vi "RoomAlert.vi"() -> ()   [LabVIEW 2018, in "Visualization.lvlib" / "VisualizeSensor.lvclass"]
doc: "This VI listens for any measurement data associated with the provided PluginName and displays it to the user for analysis. The display is only suitable for data coming from the RoomAlert Plugin."
uses:
  VisualizeSensor.lvclass
  Sensor/SensorShared/clSensorData.ctl
  <vilib>/event_ctls.llb/usereventprio.ctl
  VisualizeBase/VisualizeBase_class/Requests/VisUserEventType.ctl
  <extravilib>/ChannelInstances/Tag-bool/Write With Abort.vi
  <extravilib>/ChannelInstances/Tag-bool/Read With Abort.vi
  <extravilib>/ChannelInstances/Tag-bool/Instantiate.vi
  <extravilib>/ChannelInstances/Tag-bool/EndpointRead.vi
  <vilib>/Utility/error.llb/Error Cluster From Error Code.vi
  <extravilib>/ChannelInstances/Tag-bool/Endpoint.vi
  <vilib>/ErrorRing/Error Ring.xnode
  <userlib>/NIST/NISTErrorLib/NISTErrorLib.lvlib
  VisualizeBase/VisualizeBase_class/VisualizeBase.lvclass
  Sensor/SensorShared/SensorShared.lvlib
  Sensor/SensorModule/SensorModule.lvlib
  <extravilib>/ChannelInstances/Tag-bool.lvlib
  TestClass/Test.lvclass
panel:
  in  "ModuleID":i32
  in  "Log Data":bool=TRUE
  in  "btnStop":bool
  in  "btnReset":bool
  in  "btnClearTest":bool
  out "RoomAlert":waveform(dbl)[](graph)=[{"t0"=timestamp(3657200531.6397257 s since 1904-01-01), "dt"=1.0, "Y"=[46.19]}, {"t0"=timestamp(3657200531.6397257 s since 1904-01-01), "dt"=1.0, "Y"=[2.0]}, {"t0"=timestamp(3657200531.6397257 s since 1904-01-01), "dt"=1.0, "Y"=[60.0]}]
  out "LightTower":T1
  out "ErrorArray":errorcluster[](array[cluster])
  out "Incorrect DataType?":bool
  out "String Results":string="Sensor.RoomAlert1"
  in  "PluginName":string="Sensor.RoomAlert1"
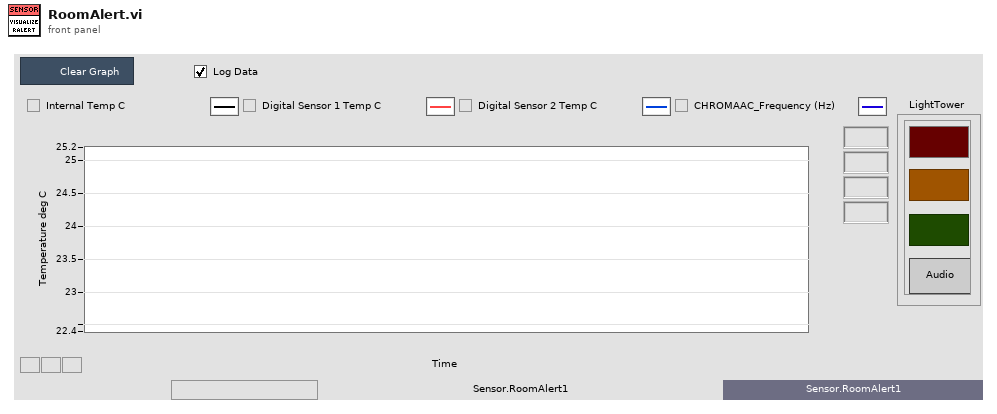
[diagram p1: front panel]
types:
  T1 = cluster{"Red":bool, "Amber":bool, "Green":bool, "Audio":bool}
  T2 = enum16{"open", "open or create", "create or replace", "create", "open (read-only)"}
  T3 = typedef "Visualization.lvlib/VisualizeBase.lvclass/VisRequestEvents.ctl" = cluster{"StopRequest":refnum<user-event>, "ResetRequest":refnum<user-event>, "FP Pop In or Out":refnum<user-event>}
  T4 = typedef "SensorShared.lvlib/clBroadcastEvents.ctl" = cluster{"DidInit":refnum<user-event>, "StatusUpdate":refnum<user-event>, "ErrorReport":refnum<user-event>, "DidStop":refnum<user-event>, "PathToINI":refnum<user-event>, "SensorReport":refnum<user-event>, "SensorConfig":refnum<user-event>}
  T5 = typedef "SensorShared.lvlib/clSensorData.ctl" = cluster{"SensorType":string, "SensorData":variant}
  T6 = typedef "Visualization.lvlib/VisualizeBase.lvclass/VisUserEventType.ctl" = cluster{"BusIndex":i8, "Data":variant}
  T7 = typedef "usereventprio.ctl" = enum32{"high priority", "normal priority"}
  T8 = cluster{"Red":bool, "Amber":bool, "Green":bool, "Audio":bool}[]
  T9 = typedef "Tag-bool.lvlib/))Channel.ctl" = refnum<queue>
  T10 = typedef "sizeaction.ctl" = enum32{"Minimized", "Maximized", "Resized"}
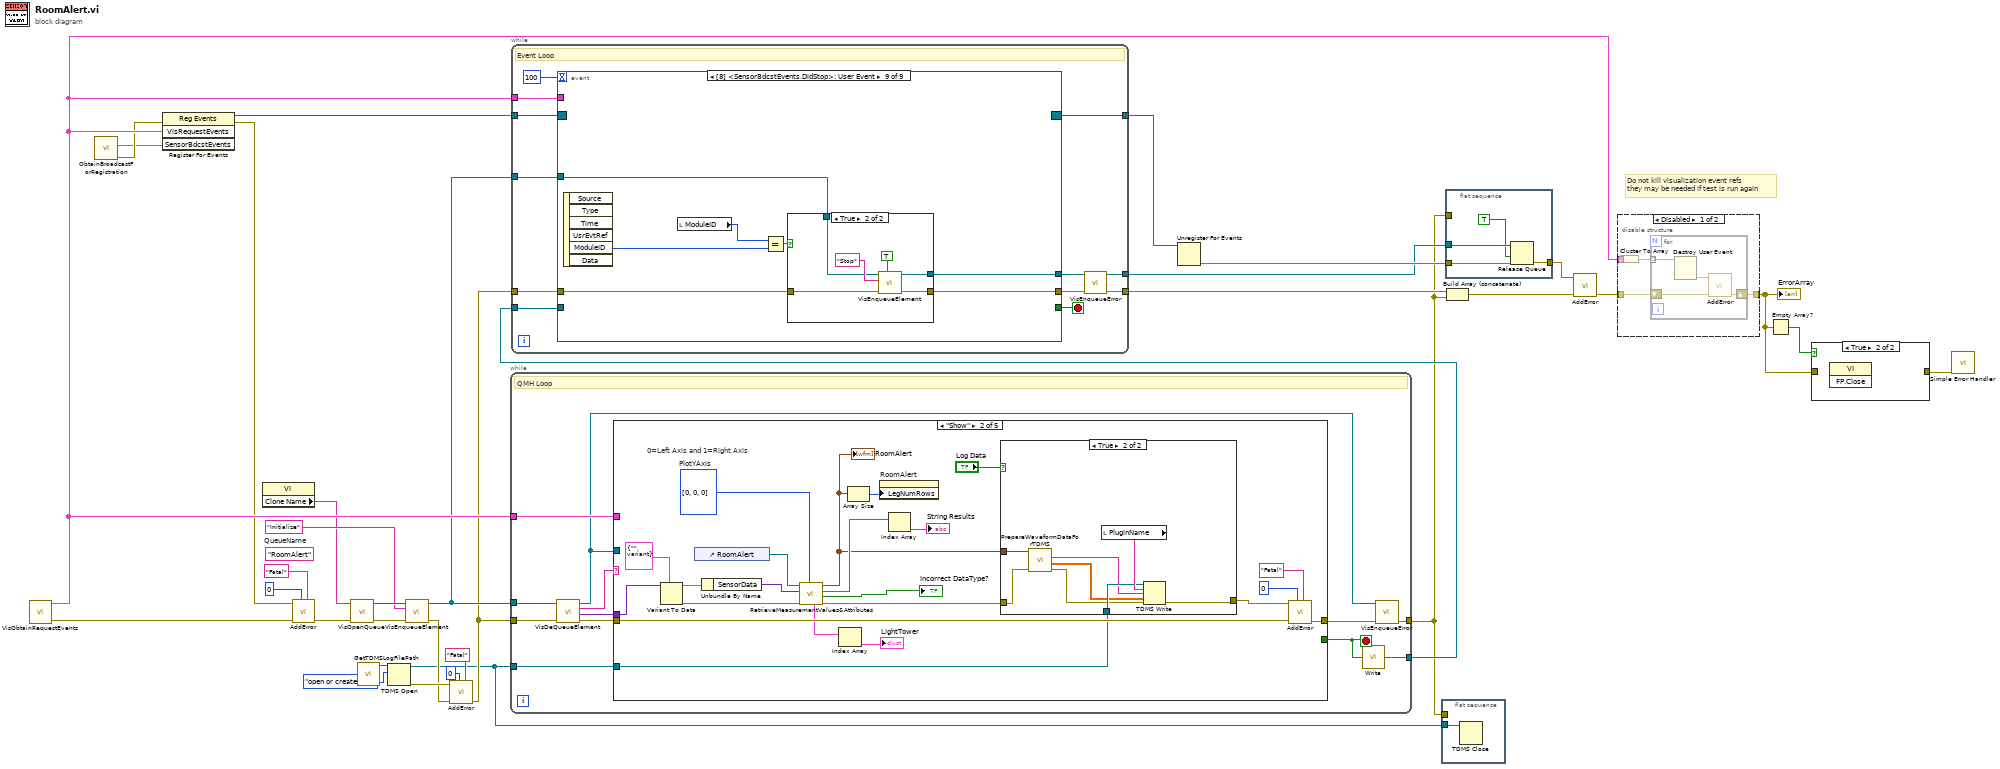
[diagram p0: block diagram]
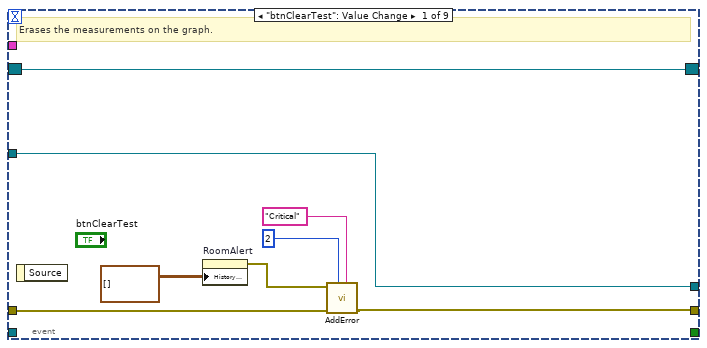
[diagram p3: hidden frame]
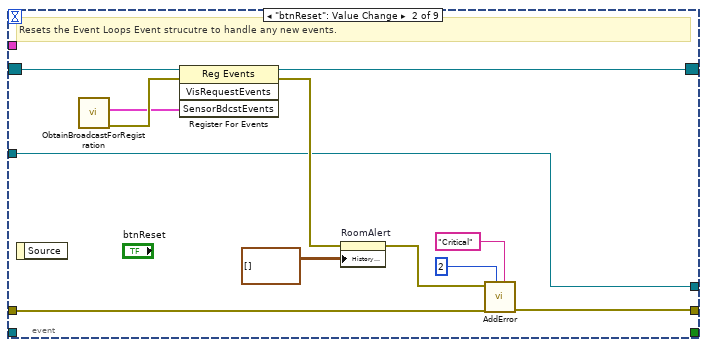
[diagram p4: hidden frame]
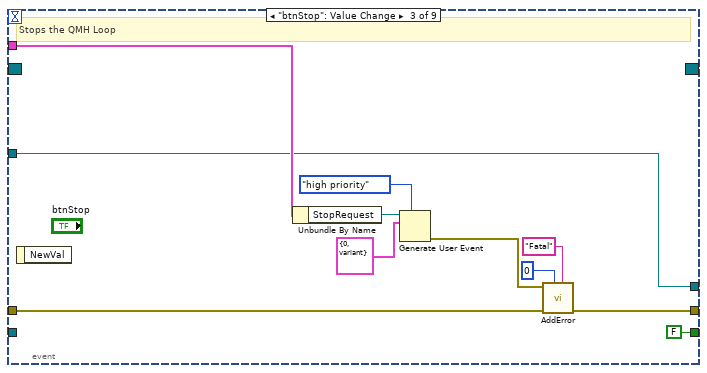
[diagram p5: hidden frame]
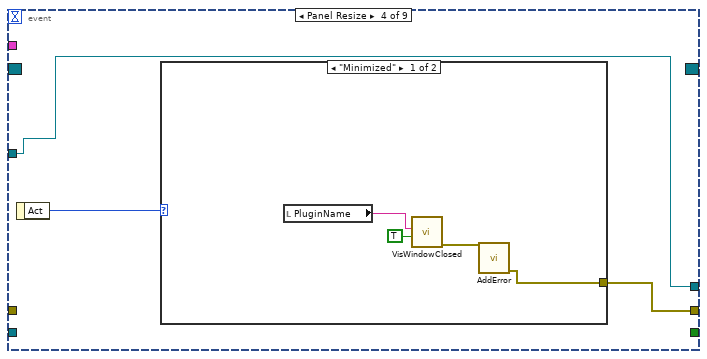
[diagram p6: hidden frame]
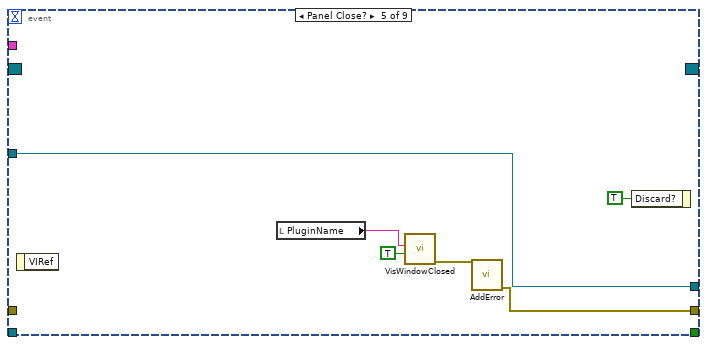
[diagram p8: hidden frame]
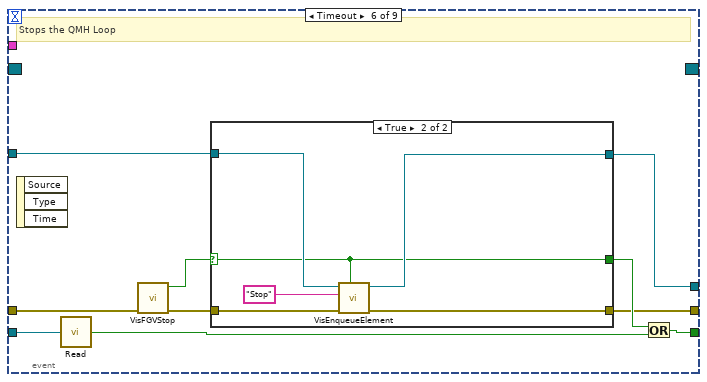
[diagram p9: hidden frame]
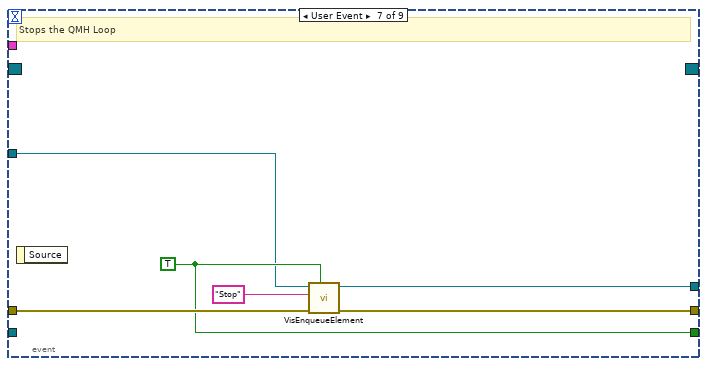
[diagram p11: hidden frame]
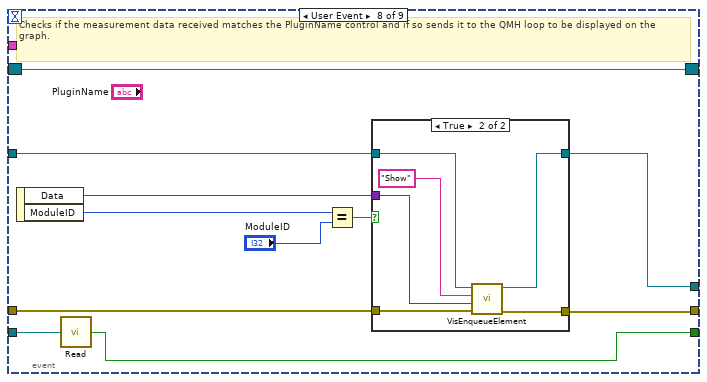
[diagram p12: hidden frame]
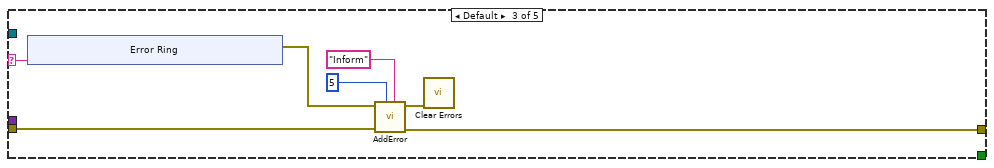
[diagram p17: hidden frame]
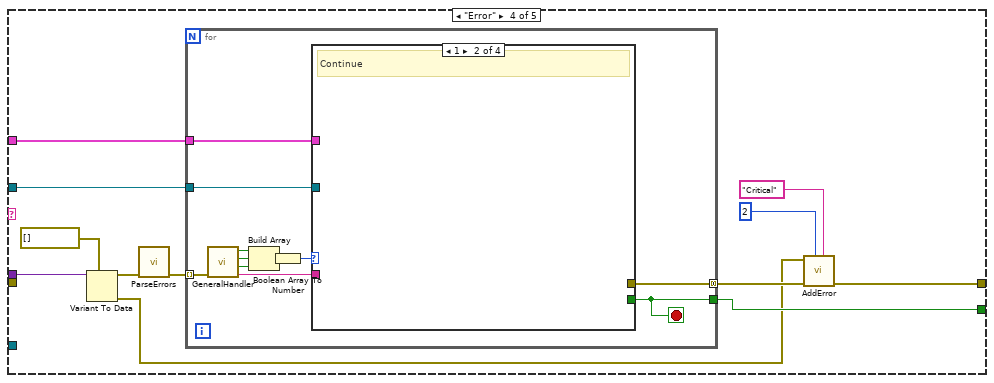
[diagram p18: hidden frame]
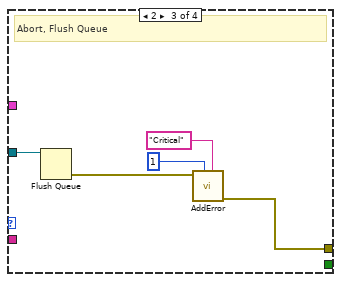
[diagram p20: hidden frame]
diagram:
  (unwired) "RoomAlert"  # QueueName
  # "Do not kill visualization event refs\nthey may be needed if test is run again"
  n1 = call "VisObtainRequestEvents.vi"() -> ("Error"=w25:errorcluster[], "VisRequestEvents"=w27:T3)  [unwired: 10 in]
  n2 = call "ObtainBroadcastForRegistration.vi"() -> ("error out"=w21:errorcluster, "SensorBdcstEvents"=w12:T4)  [unwired: 10 in]
  n3 = register-events(error in=w21, w27, w12) -> (reference out=w34:refnum<event-registration>, error out=w24:errorcluster)  [unwired: 1 in]
  n4 = property class="VI"() -> ("Clone Name"=w10:string)  [unwired: 2 in, 2 out]
  n5 = call <userlib>:"AddError.vi"("Severity"="Fatal", "Priority"=u8 0, "ErrorArray In"=w25, "error in (no error)"=w24) -> ("ErrorArray Out"=w20:errorcluster[])  [unwired: 6 in, 1 out]
  n6 = call "VisOpenQueue.vi"("Error Array In"=w20, "QueueName"=w10) -> ("Error Array Out"=w18:errorcluster[], "queue out"=w19:refnum<queue>)  [unwired: 8 in]
  n7 = call "GetTDMSLogFilePath.vi"() -> ("TDMS Log File Path"=w9:path)  [unwired: 11 in]
  n8 = TDMS Open(10:T2."open or create" ("operation (0:open)"), 11:w9) -> (0:w6:errorcluster, 3:w2:refnum<k34>)  [unwired: 5 in]
  n9 = call "VisEnqueueElement.vi"("Error Array In"=w18, "Message"="Initialize", "queue in"=w19) -> ("Error Array Out"=w5:errorcluster[], "queue out"=w16:refnum<queue>)  [unwired: 7 in]
  n10 = call <userlib>:"AddError.vi"("Severity"="Fatal", "Priority"=u8 0, "ErrorArray In"=w5, "error in (no error)"=w6) -> ("ErrorArray Out"=w4:errorcluster[])  [unwired: 6 in, 1 out]
  n11 = while {
    tunnel: w4 -> [w40]
    tunnel: [w43] -> w1
    tunnel: w16 -> [w39]
    tunnel: w27 -> [w45]
    tunnel: [w36] -> w11
    tunnel: w2 -> [w35]
    stop <- w46 stop-if-true
    # "QMH Loop"
    n12 = call "VisDeQueueElement.vi"("Error Array In"=w40, "Queue In"=w39) -> ("Error Array Out"=w38:errorcluster[], "Data"=w41:variant, "Message"=w42:string, "Queue Out"=w37:refnum<queue>)  [unwired: 6 in]
    n13 = case shown="\"Show\"" w42 {
      selector: w42 -> [_ _ w85 _ _]
      tunnel: w41 -> [_ w64 _ w104 _]
      tunnel: w38 -> [w47 w67 w83 _ w131]
      tunnel: [w47 w69 w82 w94 w131] -> w44
      tunnel: [_ _ _ w100 TRUE] -> w46
      tunnel: w45 -> [_ _ _ w99 _]
      tunnel: w37 -> [_ _ _ w98 _]
      tunnel: w35 -> [_ w55 _ _ _]
      frame "Initialize" {
      }
      frame "Show" {
        w61 = u32[] [0, 0, 0]  # PlotYAxis
        # "0=Left Axis and 1=Right Axis"
        n14 = Variant To Data(type=T5 {"SensorType"="", "SensorData"=variant} ("clSensorData"), Variant=w64) -> (data=w62:T5, error out=w63:errorcluster)  [unwired: 1 in]
        n15 = control-ref of="RoomAlert"() -> (w68:refnum<vi>)
        n16 = Unbundle By Name(w62) -> ("SensorData"=w59:variant)
        n17 = call "RetrieveMeasurementValues&Attributes.vi"("PlotYScale"=w61, "error in (no error)"=w63, "Variant"=w59, "WaveformChartReference"=w68) -> ("error out"=w58:errorcluster, "Incorrect DataType?"=→"Incorrect DataType?":bool, "Array Of Strings"=w54:string[], "WaveformArrayOut"=w48:waveform(dbl)[], "LightTower"=w52:T8)  [unwired: 3 in]
        "RoomAlert" <- w48
        n18 = Index Array(array=w52) -> (element=→"LightTower":T1)  [unwired: 1 in]
        n19 = Array Size(array=w48) -> (size(s)=w49:i32)
        n20 = property on="RoomAlert" class="WFChart (strict)"("LegNumRows"=w49) -> ()  [unwired: 2 in, 2 out]
        n21 = Index Array(array=w54) -> (element=→"String Results":string)  [unwired: 1 in]
        n22 = case shown="True" "Log Data" {
          tunnel: w58 -> [w70 w77]
          tunnel: [w70 w78] -> w57
          tunnel: w48 -> [_ w76]
          tunnel: w55 -> [_ w74]
          frame False {
          }
          frame True {
            n23 = call "PrepareWaveformDataForTDMS.vi"("error in (no error)"=w77, "WaveformArray in"=w76) -> ("error out"=w73:errorcluster, "Measurement Data"=w71:dbl[][], "Channel Names"=w72:string[])  [unwired: 7 in]
            n24 = local read "PluginName"() -> (w75:string)
            n25 = TDMS Write(0:w74, 5:w75, 7:w72, 9:w71, 11:w73) -> (15:w78:errorcluster)  [unwired: 1 in, 3 out]
          }
        }
        n26 = call <userlib>:"AddError.vi"("Severity"="Fatal" ("String"), "Priority"=u8 0, "ErrorArray In"=w67, "error in (no error)"=w57) -> ("ErrorArray Out"=w69:errorcluster[])  [unwired: 6 in, 1 out]
      }
      frame Default {
        n27 = xnode "Error Ring"("parameter 0"=w85) -> ("error out"=w84:errorcluster)
        n28 = call <userlib>:"AddError.vi"("Severity"="Inform" ("String"), "Priority"=u8 5, "ErrorArray In"=w83, "error in (no error)"=w84) -> ("ErrorArray Out"=w82:errorcluster[], "error out"=w81:errorcluster)  [unwired: 6 in]
        n29 = call <vilib>:"Clear Errors.vi"("error in (no error)"=w81) -> ()  [unwired: 5 in, 2 out]
      }
      frame "Error" {
        n30 = Variant To Data(type=errorcluster[] [], Variant=w104) -> (data=w102:errorcluster[], error out=w93:errorcluster)  [unwired: 1 in]
        n31 = call <userlib>:"ParseErrors.vi"("ErrorArray"=w102) -> ("ErrorArray"=w101:errorcluster[])  [unwired: 8 in, 2 out]
        n32 = for {
          tunnel: w101 -> [w115] mode=indexing
          tunnel: [w109] -> w95 mode=concatenating
          tunnel: [w107] -> w100
          tunnel: w99 -> [w106]
          tunnel: w98 -> [w105]
          stop <- w107 stop-if-true
          n33 = call <userlib>:"GeneralHandler.vi"("error in (no error)"=w115) -> ("Severity"=w108:string, "Stop"=w112:bool, "Abort"=w113:bool, "Continue"=w114:bool)  [unwired: 6 in, 1 out]
          n34 = Build Array(w114, w113, w112) -> (w111:bool[])
          n35 = Boolean Array To Number(Boolean array=w111) -> (number=w110:u32)
          n36 = case shown="1" w110 {
            tunnel: [_ _ w120 w129] -> w109
            tunnel: w108 -> [_ _ _ w122]
            tunnel: [_ _ _ w124] -> w107
            tunnel: w106 -> [_ _ _ w123]
            tunnel: w105 -> [_ _ w116 _]
            frame 0, Default {
              # "No Dialog"
            }
            frame 1 {
              # "Continue"
            }
            frame 2 {
              # "Abort, Flush Queue"
              n37 = Flush Queue(queue=w116) -> (error out=w119:errorcluster)  [unwired: 1 in, 2 out]
              n38 = call <userlib>:"AddError.vi"("Severity"="Critical" ("String"), "Priority"=u8 1, "error in (no error)"=w119) -> ("ErrorArray Out"=w120:errorcluster[])  [unwired: 7 in, 1 out]
            }
            frame 4 {
              # "Stop"
              n39 = Unbundle By Name(w123) -> ("StopRequest"=w130:refnum<user-event>)
              n40 = Equal?(x=w122, y="Fatal" ("x")) -> (x = y?=w124:bool)
              n41 = Generate User Event(priority (normal)=usereventprio."high priority", user event=w130, event data cluster=T6 {"BusIndex"=0, "Data"=variant} ("event data")) -> (error out=w128:errorcluster)  [unwired: 1 in, 1 out]
              n42 = call <userlib>:"AddError.vi"("error in (no error)"=w128) -> ("ErrorArray Out"=w129:errorcluster[], "error out"=w125:errorcluster)  [unwired: 9 in]
              n43 = call <vilib>:"Clear Errors.vi"("error in (no error)"=w125) -> ()  [unwired: 5 in, 2 out]
            }
          }
        }
        n44 = call <userlib>:"AddError.vi"("Severity"="Critical", "Priority"=u8 2, "ErrorArray In"=w95, "error in (no error)"=w93) -> ("ErrorArray Out"=w94:errorcluster[])  [unwired: 6 in, 1 out]
      }
      frame "Stop" {
      }
    }
    n45 = call <extravilib>:"Write.vi"("element"=w46) -> ("channel"=w36:T9)  [unwired: 1 out]
    n46 = call "VisEnqueueError.vi"("Error Array In"=w44, "Queue in"=w37) -> ("Error Array Out"=w43:errorcluster[])  [unwired: 8 in, 1 out]
  }
  n47 = while {
    tunnel: w34 -> [w144]
    tunnel: [w138] -> w32
    tunnel: [w142] -> w33
    tunnel: w27 -> [w141]
    tunnel: w4 -> [w140]
    tunnel: w16 -> [w139]
    tunnel: [w135] -> w15
    tunnel: w11 -> [w133]
    stop <- w143 stop-if-true
    # "Event Loop"
    n48 = event shown="[8] <SensorBdcstEvents.DidStop>: User Event" {
      selector: w144 -> [w146 w164 _ _ _ _ _ w220 _]
      dyn-events: [w146 w163 _ _ _ _ _ w220 _] -> w142
      timeout: 100 -> [_ _ _ _ _ _ _ _ _]
      tunnel: [_ _ FALSE ("Priority? (F)") _ _ w189 w210 w217 _] -> w143
      tunnel: [w149 w161 w168 w177 w184 w191 w212 w222 w236] -> w137
      tunnel: w141 -> [_ _ w167 _ _ _ _ _ _]
      tunnel: w140 -> [w150 w162 w175 _ _ w194 w213 w223 w235]
      tunnel: w139 -> [w145 w154 w165 w176 w183 w193 w208 w224 w238]
      tunnel: [w145 w154 w165 w176 w183 w192 w211 w221 w237] -> w136
      tunnel: w133 -> [_ _ _ _ _ w198 _ w218 _]
      event "btnClearTest": Value Change {
        # "Erases the measurements on the graph."
        n49 = event-data() -> ()  [unwired: 1 in, 1 out]
        n50 = property on="RoomAlert" class="WFChart (strict)"("History Data"=waveform(dbl)[][] []) -> (error out=w148:errorcluster)  [unwired: 2 in, 1 out]
        n51 = call <userlib>:"AddError.vi"("Severity"="Critical", "Priority"=u8 2, "ErrorArray In"=w150, "error in (no error)"=w148) -> ("ErrorArray Out"=w149:errorcluster[])  [unwired: 6 in, 1 out]
      }
      event "btnReset": Value Change {
        # "Resets the Event Loops Event strucutre to handle any new events."
        n52 = event-data() -> ()  [unwired: 1 in, 1 out]
        n53 = call "ObtainBroadcastForRegistration.vi"() -> ("error out"=w155:errorcluster, "SensorBdcstEvents"=w153:T4)  [unwired: 10 in]
        n54 = register-events(reference=w164, error in=w155, w153) -> (reference out=w163:refnum<event-registration>, error out=w157:errorcluster)  [unwired: 1 in]
        n55 = property on="RoomAlert" class="WFChart (strict)"(error in=w157, "History Data"=waveform(dbl)[][] []) -> (error out=w156:errorcluster)  [unwired: 1 in, 1 out]
        n56 = call <userlib>:"AddError.vi"("Severity"="Critical", "Priority"=u8 2, "ErrorArray In"=w162, "error in (no error)"=w156) -> ("ErrorArray Out"=w161:errorcluster[])  [unwired: 6 in, 1 out]
      }
      event "btnStop": Value Change {
        # "Stops the QMH Loop"
        n57 = event-data() -> ()  [unwired: 1 in, 1 out]
        n58 = Unbundle By Name(w167) -> ("StopRequest"=w173:refnum<user-event>)
        n59 = Generate User Event(priority (normal)=usereventprio."high priority", user event=w173, event data cluster=T6 {"BusIndex"=0, "Data"=variant} ("event data")) -> (error out=w174:errorcluster)  [unwired: 1 in, 1 out]
        n60 = call <userlib>:"AddError.vi"("Severity"="Fatal" ("String"), "Priority"=u8 0, "ErrorArray In"=w175, "error in (no error)"=w174) -> ("ErrorArray Out"=w168:errorcluster[])  [unwired: 6 in, 1 out]
      }
      event Panel Resize {
        n61 = event-data() -> ("Act"=w178:T10)  [unwired: 1 in]
        n62 = case shown="\"Minimized\"" w178 {
          tunnel: [w179 _] -> w177
          frame "Minimized" {
            n63 = local read "PluginName"() -> (w181:string)
            n64 = call "VisWindowClosed.vi"("Window Closed?"=TRUE ("Window Minimized or Clozed?"), "Module Name"=w181) -> ("error out"=w182:errorcluster)  [unwired: 9 in]
            n65 = call <userlib>:"AddError.vi"("error in (no error)"=w182) -> ("ErrorArray Out"=w179:errorcluster[])  [unwired: 9 in, 1 out]
          }
          frame "Maximized", Default {
          }
        }
      }
      event Panel Close? {
        n66 = event-data() -> ()  [unwired: 1 in, 1 out]
        n67 = local read "PluginName"() -> (w185:string)
        n68 = call "VisWindowClosed.vi"("Window Closed?"=TRUE ("Window Minimized or Clozed?"), "Module Name"=w185) -> ("error out"=w186:errorcluster)  [unwired: 9 in]
        n69 = call <userlib>:"AddError.vi"("error in (no error)"=w186) -> ("ErrorArray Out"=w184:errorcluster[])  [unwired: 9 in, 1 out]
        n70 = event-data("Discard?"=TRUE) -> ()  [unwired: 1 in, 1 out]
      }
      event Timeout {
        # "Stops the QMH Loop"
        n71 = event-data() -> ()  [unwired: 1 in, 3 out]
        n72 = call <extravilib>:"Read.vi"("channel"=w198) -> ("element"=w190:bool)  [unwired: 1 in, 1 out]
        n73 = call "VisFGVStop.vi"("Error In"=w194) -> ("Error Out"=w196:errorcluster[], "Value"=w197:bool)  [unwired: 9 in]
        n74 = case shown="True" w197 {
          selector: w197 -> [w199 w202]
          tunnel: [w201 w205] -> w191
          tunnel: w196 -> [w201 w206]
          tunnel: w193 -> [w200 w204]
          tunnel: [w200 w203] -> w192
          tunnel: [w199 w202] -> w195
          frame False {
          }
          frame True {
            n75 = call "VisEnqueueElement.vi"("Priority? (F)"=w202, "Error Array In"=w206, "Message"="Stop", "queue in"=w204) -> ("Error Array Out"=w205:errorcluster[], "queue out"=w203:refnum<queue>)  [unwired: 6 in]
          }
        }
        n76 = Or(x=w195, y=w190) -> (x .or. y?=w189:bool)
      }
      event User Event {
        w210 = TRUE ("Priority? (F)")
        # "Stops the QMH Loop"
        n77 = event-data() -> ()  [unwired: 1 in, 1 out]
        n78 = call "VisEnqueueElement.vi"("Priority? (F)"=w210, "Error Array In"=w213, "Message"="Stop", "queue in"=w208) -> ("Error Array Out"=w212:errorcluster[], "queue out"=w211:refnum<queue>)  [unwired: 6 in]
      }
      event User Event {
        # "Checks if the measurement data received matches the PluginName control and if so sends it to the QMH loop to be displayed on the graph."
        n79 = event-data() -> ("Data"=w219:variant, "ModuleID"=w214:i32)  [unwired: 1 in]
        n80 = call <extravilib>:"Read.vi"("channel"=w218) -> ("element"=w217:bool)  [unwired: 1 in, 1 out]
        n81 = Equal?(x=w214, y="ModuleID") -> (x = y?=w216:bool)
        n82 = case shown="True" w216 {
          tunnel: [w225 w231] -> w222
          tunnel: w224 -> [w226 w230]
          tunnel: w223 -> [w225 w232]
          tunnel: [w226 w228] -> w221
          tunnel: w219 -> [_ w229]
          frame False {
          }
          frame True {
            n83 = call "VisEnqueueElement.vi"("Error Array In"=w232, "Data"=w229, "Message"="Show", "queue in"=w230) -> ("Error Array Out"=w231:errorcluster[], "queue out"=w228:refnum<queue>)  [unwired: 6 in]
          }
        }
      }
      event User Event {
        n84 = event-data() -> ("ModuleID"=w234:i32)  [unwired: 1 in, 5 out]
        n85 = local read "ModuleID"() -> (w233:i32)
        n86 = Equal?(x=w233, y=w234) -> (x = y?=w239:bool)
        n87 = case shown="True" w239 {
          tunnel: [w240 w245] -> w236
          tunnel: [w241 w244] -> w237
          tunnel: w238 -> [w241 w243]
          tunnel: w235 -> [w240 w242]
          frame False {
          }
          frame True {
            n88 = call "VisEnqueueElement.vi"("Priority? (F)"=TRUE, "Error Array In"=w242, "Message"="Stop", "queue in"=w243) -> ("Error Array Out"=w245:errorcluster[], "queue out"=w244:refnum<queue>)  [unwired: 6 in]
          }
        }
      }
    }
    n89 = call "VisEnqueueError.vi"("Error Array In"=w137, "Queue in"=w136) -> ("Error Array Out"=w138:errorcluster[], "Queue out"=w135:refnum<queue>)  [unwired: 8 in]
  }
  n90 = Unregister For Events(event registration refnum=w33) -> (error out=w31:errorcluster)  [unwired: 1 in]
  n91 = flat-sequence {
    tunnel: w2 -> [w248]
    tunnel: w1 -> [_]
    frame #0 {
      n92 = TDMS Close(11:w248) -> ()  [unwired: 1 in, 2 out]
    }
  }
  n93 = flat-sequence {
    tunnel: w31 -> [w252]
    tunnel: [w251] -> w29
    tunnel: w15 -> [w250]
    tunnel: w1 -> [_]
    frame #0 {
      n94 = Release Queue(queue=w250, force destroy? (F)=TRUE, error in (no error)=w252) -> (error out=w251:errorcluster)  [unwired: 2 out]
    }
  }
  n95 = Build Array (concatenate)(w32, w1) -> (w30:errorcluster[])
  n96 = call <userlib>:"AddError.vi"("ErrorArray In"=w30, "error in (no error)"=w29) -> ("ErrorArray Out"=w28:errorcluster[])  [unwired: 8 in, 1 out]
  n97 = disable-structure shown="Disabled" {
    disable-tunnel: w28 -> [w255 w261]
    disable-tunnel: w27 -> [w254 _]
    disable-tunnel: [w253 w261] -> w14
    frame Disabled {
      n98 = Cluster To Array(cluster=w254) -> (array=w256:refnum<user-event>[])
      n99 = for {
        tunnel: w256 -> [w260] mode=indexing
        shift-right: [w259] -> w253
        shift-left: w255 -> [w258]
        n100 = Destroy User Event(user event=w260) -> (error out=w257:errorcluster)  [unwired: 1 in]
        n101 = call <userlib>:"AddError.vi"("ErrorArray In"=w258, "error in (no error)"=w257) -> ("ErrorArray Out"=w259:errorcluster[])  [unwired: 8 in, 1 out]
      }
    }
    frame Enabled {
    }
  }
  "ErrorArray" <- w14
  n102 = Empty Array?(array=w14) -> (empty?=w26:bool)
  n103 = case shown="True" w26 {
    tunnel: [w262 _] -> w13
    tunnel: w14 -> [w263 _]
    frame False {
      n104 = Merge Errors(w263) -> (w262:errorcluster)
    }
    frame True {
      n105 = invoke class="VI" method="FP.Close"() -> ()  [unwired: 3 in, 3 out]
    }
  }
  n106 = call <vilib>:"Simple Error Handler.vi"("error in (no error)"=w13) -> ()  [unwired: 4 in, 5 out]
